vi "splitArea.vi"(11 "InfoMissao":T1 {"Agentes Disponíveis" format="%#_13g"}) -> (3 "Array":dbl[](array[numeric]))   [LabVIEW 2018]
uses:
  InfoMissao.ctl
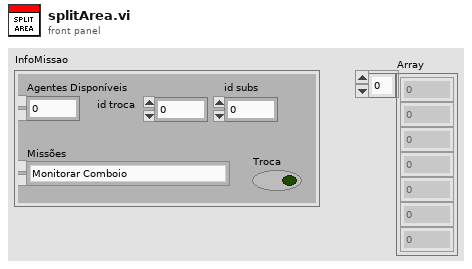
[diagram p1: front panel]
types:
  T1 = typedef "InfoMissao.ctl" = cluster{"Troca ":bool, "Missões ":enum16{"Monitorar Comboio", "Realizar Segurança de Retaguarda", "Vigiar Área", "Reconhecimento de Área"}, "Agentes Disponíveis":dbl, "id troca ":dbl, "id subs":dbl}
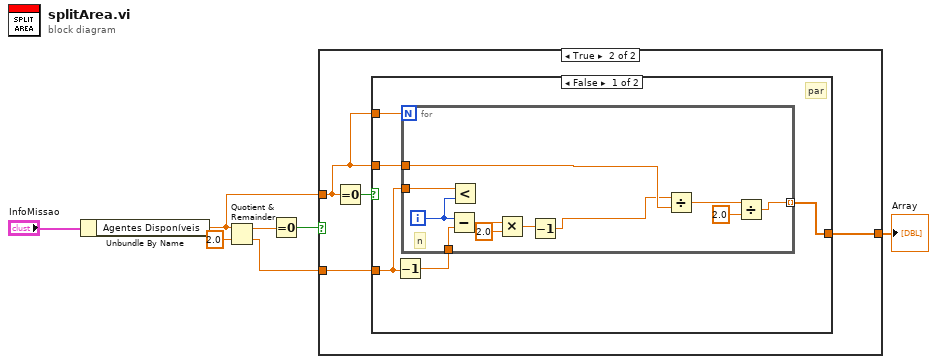
[diagram p0: block diagram]
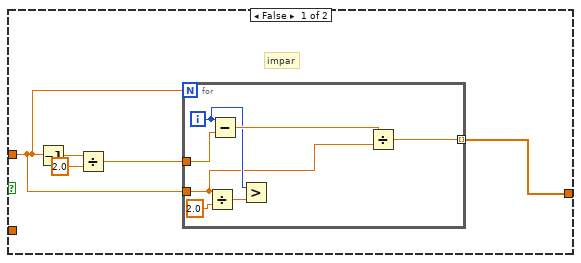
[diagram p2: hidden frame]
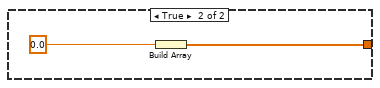
[diagram p3: hidden frame]
diagram:
  n1 = Unbundle By Name("InfoMissao") -> ("Agentes Disponíveis"=w3:dbl)
  n2 = Quotient & Remainder(x=w3, y=2.0) -> (x-y*floor(x/y)=w4:dbl, floor(x/y)=w2:dbl)
  n3 = Equal To 0?(x=w4) -> (x = 0?=w5:bool)
  n4 = case shown="True" w5 {
    tunnel: w3 -> [w8 w20]
    tunnel: [w9 w22] -> w1
    tunnel: w2 -> [_ w21]
    frame False {
      # "impar"
      n5 = Decrement(x=w8) -> (x-1=w12:dbl)
      n6 = Divide(x=w12, y=2.0) -> (x/y=w10:dbl)
      n7 = for {
        N: w8 -> [_]
        tunnel: w10 -> [w19]
        tunnel: w8 -> [w14]
        tunnel: [w13] -> w9 mode=indexing
        i -> [w15]
        n8 = Divide(x=w14, y=2.0) -> (x/y=w16:dbl)
        n9 = Subtract(x=w15, y=w19) -> (x-y=w18:dbl)
        n10 = Greater?(x=w15, y=w16) -> ()  [unwired: 1 out]
        n11 = Divide(x=w18, y=w14) -> (x/y=w13:dbl)
      }
    }
    frame True {
      n12 = Equal To 0?(x=w20) -> (x = 0?=w23:bool)
      n13 = case shown="False" w23 {
        tunnel: [w25 w40] -> w22
        tunnel: w21 -> [w27 _]
        tunnel: w20 -> [w26 _]
        tunnel: w20 -> [w24 _]
        frame False {
          # "par"
          n14 = Decrement(x=w27) -> (x-1=w28:dbl)
          n15 = for {
            N: w24 -> [_]
            tunnel: w28 -> [w39]
            tunnel: w27 -> [w37]
            tunnel: w26 -> [w36]
            tunnel: [w30] -> w25 mode=indexing
            i -> [w38]
            # "n"
            n16 = Subtract(x=w38, y=w39) -> (x-y=w35:dbl)
            n17 = Less?(x=w37, y=w38) -> ()  [unwired: 1 out]
            n18 = Multiply(x=w35, y=2.0) -> (x*y=w33:dbl)
            n19 = Decrement(x=w33) -> (x-1=w32:dbl)
            n20 = Divide(x=w32, y=w36) -> (x/y=w31:dbl)
            n21 = Divide(x=w31, y=2.0) -> (x/y=w30:dbl)
          }
        }
        frame True {
          n22 = Build Array(0.0) -> (w40:dbl[])
        }
      }
    }
  }
  "Array" <- w1
